vi "Create CLI Input Summary String.vi"(11 "CLI Inputs":T1) -> (3 "Summary String":string)   [LabVIEW 2019]
uses:
  CLI-Inputs.ctl
  TargetType.ctl
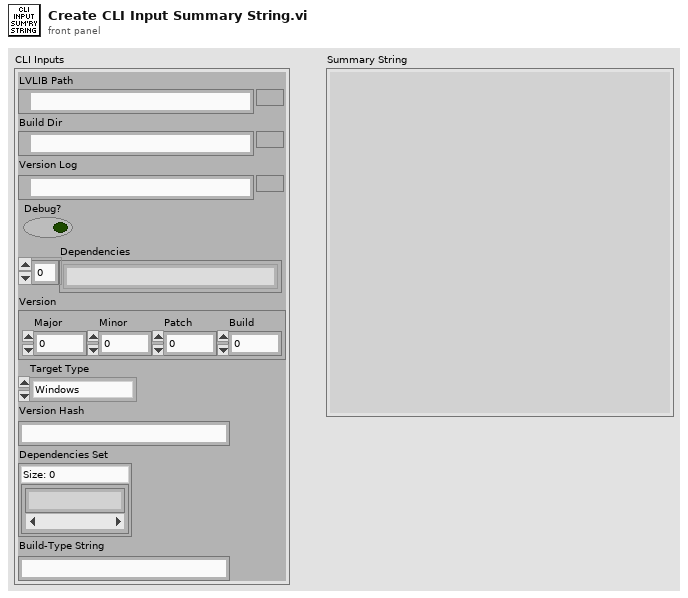
[diagram p1: front panel]
types:
  T1 = typedef "CLI-Inputs.ctl" = cluster{"LVLIB Path":path, "Build Dir":path, "VersionLog":path, "Debug?":bool, "Dependencies":string[], "Version":cluster{"Major":i32, "Minor":i32, "Patch":i32, "Build":i32}, "Target Type":T2, "Version Hash":string, "Dependencies Set":set{string}, "Build Type":string}
  T2 = typedef "TargetType.ctl" = enum16{"Windows", "cRIO-9045"}
  T3 = cluster{"Major":i32, "Minor":i32, "Patch":i32, "Build":i32}
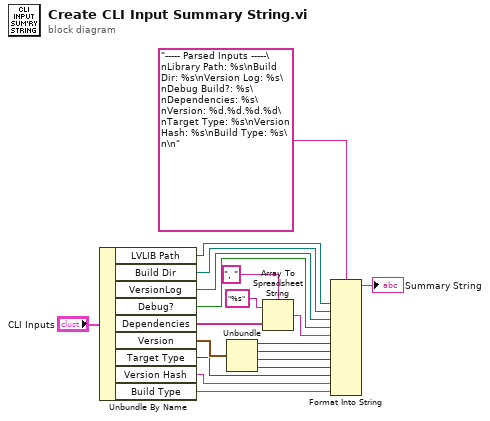
[diagram p0: block diagram]
diagram:
  n1 = Unbundle By Name("CLI Inputs") -> ("LVLIB Path"=w14:path, "Build Dir"=w13:path, "VersionLog"=w12:path, "Debug?"=w11:bool, "Dependencies"=w10:string[], "Version"=w8:T3, "Target Type"=w3:T2, "Version Hash"=w2:string, "Build Type"=w1:string)
  n2 = Unbundle(w8) -> ("Major"=w7:i32, "Minor"=w6:i32, "Patch"=w5:i32, "Build"=w4:i32)
  n3 = Array To Spreadsheet String(delimiter (Tab)=", ", array=w10, 3:"%s" ("format string")) -> (spreadsheet string=w9:string)
  n4 = Format Into String(format string="----- Parsed Inputs -----\nLibrary Path: %s\nBuild Dir: %s\nVersion Log: %s\nDebug Build?: %s\nDependencies: %s\nVersion: %d.%d.%d.%d\nTarget Type: %s\nVersion Hash: %s\nBuild Type: %s\n\n", w14, w13, w12, w11, w9, w7, w6, w5, w4, w3, w2, w1) -> (resulting string=→"Summary String":string)  [unwired: 2 in, 1 out]
